vi "Temperature Control.vi"(8 "error in (no error)":errorcluster, 10 "Temperature Controller.lvclass":refnum<class "Temperature Controller.lvclass">, 11 "Temperature Control.lvclass":refnum<class "Temperature Control.lvclass">) -> (0 "error out":errorcluster, 3 "Reader out":refnum<class "Temperature Control.lvclass">)   [LabVIEW 2009, in "Temperature Control.lvclass"]
uses:
  Temperature Control.lvclass
  Instruments/Magnet/Temperature Controller/Temperature Controller.lvclass
  Reader/Reader.lvclass
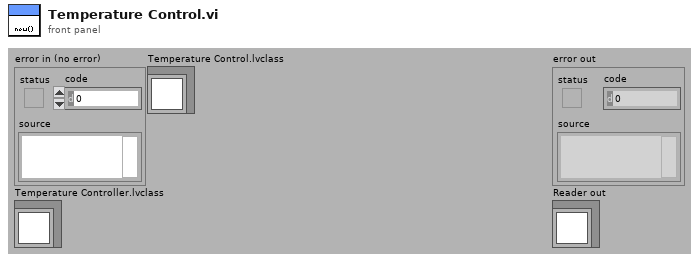
[diagram p1: front panel]
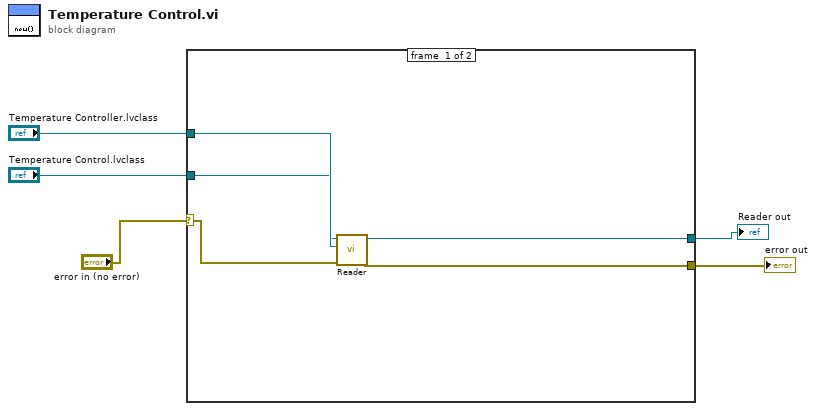
[diagram p0: block diagram]
diagram:
  n1 = case shown="No Error" "error in (no error)" {
    selector: "error in (no error)" -> [w10 w12]
    tunnel: "Temperature Controller.lvclass" -> [w9 _]
    tunnel: [w8 w12] -> w3
    tunnel: "Temperature Control.lvclass" -> [w7 w11]
    tunnel: [w6 w11] -> w1
    frame #0 {
      n2 = call "Reader.vi"("error in (no error)"=w10, "Readable"=w9, "Reader in"=w7) -> ("error out"=w8:errorcluster, "Reader out"=w6:refnum<class "Temperature Control.lvclass">)  [unwired: 7 out]
    }
    frame #1 {
    }
  }
  "error out" <- w3
  "Reader out" <- w1
